vi "Dispatch Get Metadata Async.vi"(8 "error in (no error)":errorcluster, 10 "measurement plugin service in":refnum<class "Measurement Plugin Service.lvclass">, 11 "gRPC ID in":T1) -> (0 "error out":errorcluster)   [LabVIEW 2021, in "NI Measurement Plug-In SDK.lvlib" / "Measurement Service V2.lvclass"]
uses:
  Measurement Service V2.lvclass
  <vilib>/gRPC/LabVIEW gRPC Library/Shared/grpcId.ctl
  Measurement Plugin Service/Measurement Plugin Service.lvclass
  Handle Get Metadata RPC.vi
  IMeasurement Service/IMeasurement Service.lvclass
  <vilib>/gRPC/LabVIEW gRPC Library/grpc-lvsupport-release.lvlib
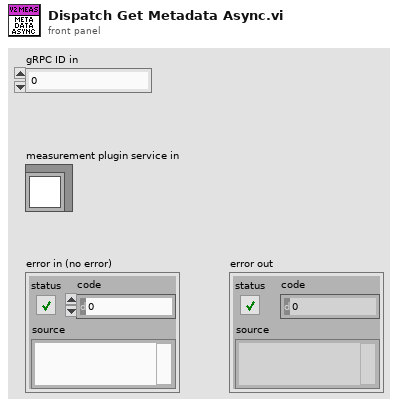
[diagram p1: front panel]
types:
  T1 = typedef "grpc-lvsupport-release.lvlib/grpcId.ctl" = u64
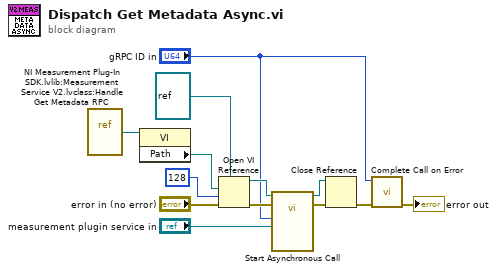
[diagram p0: block diagram]
diagram:
  n1 = vi-ref "NI Measurement Plug-In SDK.lvlib:Measurement Service V2.lvclass:Handle Get Metadata RPC.vi"() -> (w2:refnum<vi>)
  n2 = property class="VI"(reference=w2) -> ("Path"=w1:path)  [unwired: 1 in, 2 out]
  n3 = Open VI Reference(type specifier VI Refnum (for type only)=refnum<vi> refnum, vi path=w1, options=128, error in (no error)="error in (no error)") -> (vi reference=w11:refnum<vi>, error out=w10:errorcluster)  [unwired: 2 in]
  n4 = call-by-ref "Start Asynchronous Call"(reference=w11, error in=w10, "measurement plugin service in"="measurement plugin service in", "gRPC ID"="gRPC ID in") -> (reference out=w3:refnum<vi>, error out=w4:errorcluster)  [unwired: 10 in]
  n5 = Close Reference(reference=w3, error in (no error)=w4) -> (error out=w5:errorcluster)
  n6 = call "Complete Call on Error.vi"("error in"=w5, "gRPC ID in"="gRPC ID in") -> ("error out"=→"error out":errorcluster)  [unwired: 9 in]
